vi "Get Module Execution Status by ref.vi"(8 "Modules Tree ref":refnum<vi>, 11 "Helper Loop Cluster":T1) -> (0 "error out":errorcluster)   [LabVIEW 2020, in "Panther Dashboard.lvlib"]
doc: "This VI checks the Main.vi State of the selected DQMH Module"
uses:
  Panther Dashboard.lvlib
  Helper Loop--cluster.ctl
  Module type--enum.ctl
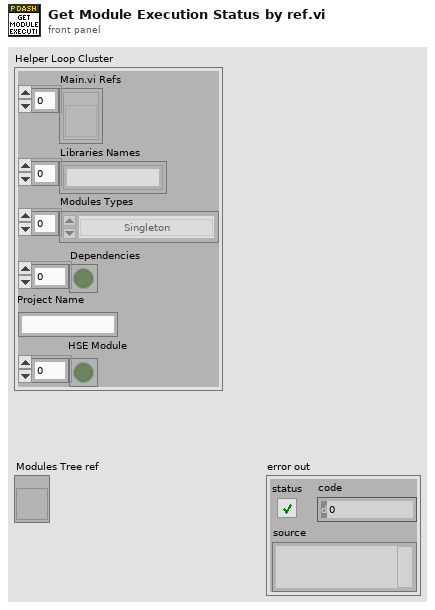
[diagram p1: front panel]
types:
  T1 = typedef "Panther Dashboard.lvlib/Helper Loop--cluster.ctl" = cluster{"Main.vi Refs":refnum<vi>[], "Libraries Names":string[], "Modules Types":T2[], "Dependencies":bool[], "Project Name":string, "HSE Module":bool[]}
  T2 = typedef "Panther Dashboard.lvlib/Module type--enum.ctl" = enum16{"Singleton", "Cloneable"}
  T3 = enum32{"Bad", "Idle", "Run top level", "Running"}
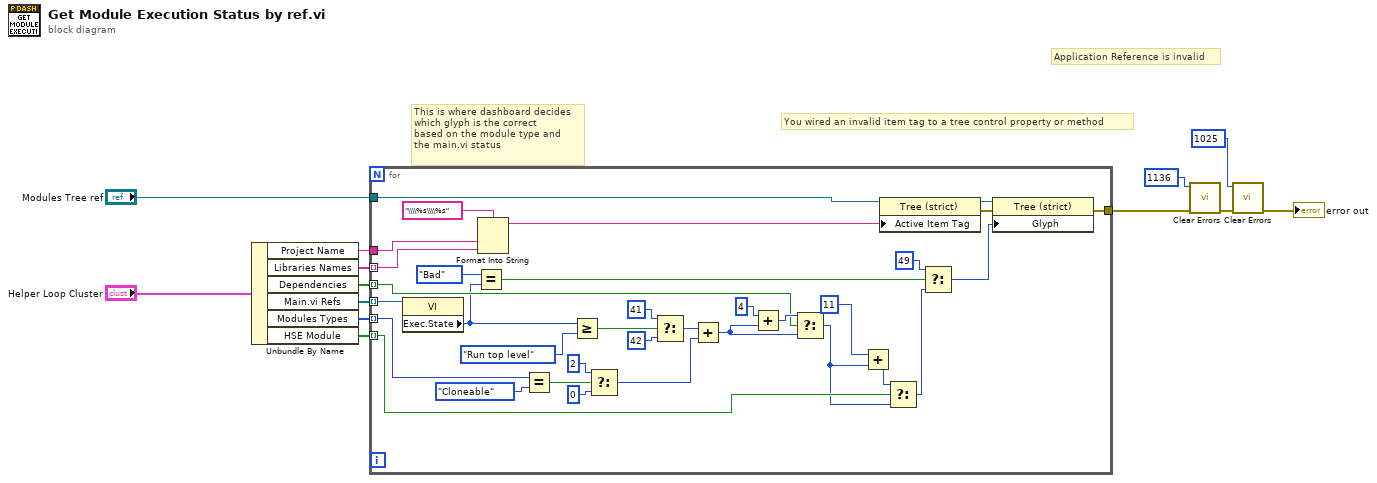
[diagram p0: block diagram]
diagram:
  # "This is where dashboard decides\nwhich glyph is the correct\nbased on the module type and\nthe main.vi status"
  # "Application Reference is invalid"
  # "You wired an invalid item tag to a tree control property or method"
  n1 = Unbundle By Name("Helper Loop Cluster") -> ("Project Name"=w2:string, "Libraries Names"=w6:string[], "Dependencies"=w5:bool[], "Main.vi Refs"=w4:refnum<vi>[], "Modules Types"=w3:T2[], "HSE Module"=w1:bool[])
  n2 = for {
    tunnel: [w46] -> w10
    tunnel: "Modules Tree ref" -> [w44]
    tunnel: w3 -> [w36] mode=indexing
    tunnel: w5 -> [w28] mode=indexing
    tunnel: w4 -> [w25] mode=indexing
    tunnel: w6 -> [w26] mode=indexing
    tunnel: w2 -> [w19]
    tunnel: w1 -> [w18] mode=indexing
    n3 = property class="VI"(reference=w25) -> ("Exec.State"=w21:T3)  [unwired: 1 in, 2 out]
    n4 = Equal?(x=T3."Bad" ("y"), y=w21) -> (x = y?=w22:bool)
    n5 = Format Into String(format string="\\\\%s\\\\%s", w19, w26) -> (resulting string=w43:string)  [unwired: 2 in, 1 out]
    n6 = Equal?(x=w36, y=Module_type--enum."Cloneable" ("x")) -> (x = y?=w34:bool)
    n7 = Greater Or Equal?(x=w21, y=T3."Run top level") -> (x >= y?=w39:bool)
    n8 = Select(t=2, s=w34, f=0) -> (s? t:f=w31:i32)
    n9 = Select(t=41, s=w39, f=42) -> (s? t:f=w41:i32)
    n10 = Add(x=w41, y=w31) -> (x+y=w27:i32)
    n11 = Add(x=4 ("y"), y=w27) -> (x+y=w29:i32)
    n12 = Select(t=w29, s=w28, f=w27) -> (s? t:f=w15:i32)
    n13 = Add(x=11, y=w15) -> (x+y=w16:i32)
    n14 = property class="Tree (strict)"(reference=w44, "Active Item Tag"=w43) -> (reference out=w42:refnum<vi>, error out=w47:errorcluster)  [unwired: 1 in]
    n15 = Select(t=w16, s=w18, f=w15) -> (s? t:f=w17:i32)
    n16 = Select(t=49 ("y"), s=w22, f=w17) -> (s? t:f=w24:i32)
    n17 = property class="Tree (strict)"(reference=w42, error in=w47, "Glyph"=w24) -> (error out=w46:errorcluster)  [unwired: 1 out]
  }
  n18 = call <vilib>:"Clear Errors.vi"("error in (no error)"=w10, "specific error code to clear (0: all)"=1136) -> ("error out"=w9:errorcluster)  [unwired: 4 in, 1 out]
  n19 = call <vilib>:"Clear Errors.vi"("error in (no error)"=w9, "specific error code to clear (0: all)"=1025) -> ("error out"=→"error out":errorcluster)  [unwired: 4 in, 1 out]
